vi "ParseFloatChannel.vi"(11 "Input":string) -> (3 "Array":dbl[](array[numeric]))   [LabVIEW 2019]
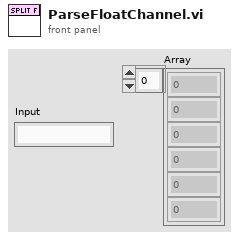
[diagram p1: front panel]
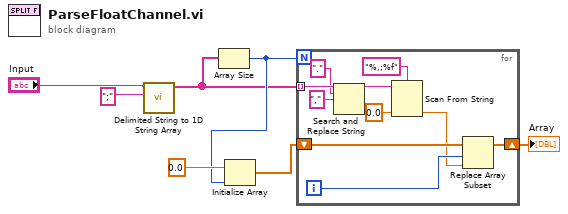
[diagram p0: block diagram]
diagram:
  n1 = call <vilib>:"Delimited String to 1D String Array.vi"("delimiter"=";" ("search string/char (-)"), "delimited string"="Input") -> ("string array"=w3:string[])  [unwired: 9 in]
  n2 = Array Size(array=w3) -> (size(s)=w4:i32)
  n3 = Initialize Array(0.0, w4) -> (w1:dbl[])
  n4 = for {
    N: w4 -> [_]
    tunnel: w3 -> [w14] mode=indexing
    shift-right: [w16] -> w2
    shift-left: w1 -> [w15]
    i -> [w17]
    n5 = Search and Replace String(input string=w14, search string=".", replace string="," ("replace string (\"\")")) -> (result string=w11:string)  [unwired: 5 in, 3 out]
    n6 = Scan From String(format string="%,;%f", input string=w11, default 1=0.0 ("default value 1")) -> (output 1=w10:dbl)  [unwired: 2 in, 3 out]
    n7 = Replace Array Subset(array=w15, new element=w10, index=w17) -> (w16:dbl[])
  }
  "Array" <- w2
